vi "GetSettings.vi"(8 "error in (no error)":errorcluster, 10 "SettingsToRetrieve":variant, 11 "NHRDCPower in":refnum<class "NHRDCPower.lvclass">) -> (0 "error out":errorcluster, 2 "RetrievedSettings":variant, 3 "NHRDCPower Out":refnum<class "NHRDCPower.lvclass">)   [LabVIEW 2018, in "AcPwrPlugins.lvlib" / "NHRDCPower.lvclass"]
doc: "This VI retrieves a boolean status to see if the instrument can conduct measurements while the device is changing modes or turning off and on."
uses:
  NHRDCPower.lvclass
  C:/Users/ico/Documents/Projects/NistPluggableModules/AcPwr/AcPwrPlugins/AcPwrBaseClass/AcPwrBase.lvclass
  AcPwrBaseClass/AcPwrBase.lvclass/AcPwrBase.ctl
  AcPwrBaseClass/TypeDefs/BaseMeasurements.ctl
  ChromaAcLoad/TypeDefs/MeasurementType.ctl
  AcPwrBaseClass/Accessors/Read BaseConfig.vi
  AcPwrModule/AcPwrModule.lvlib
  ChromaAcLoad/ChromaAcLoad.lvclass
  AcPwrBaseClass/AcPwrBase.lvclass
panel:
  out "Boolean":bool=TRUE
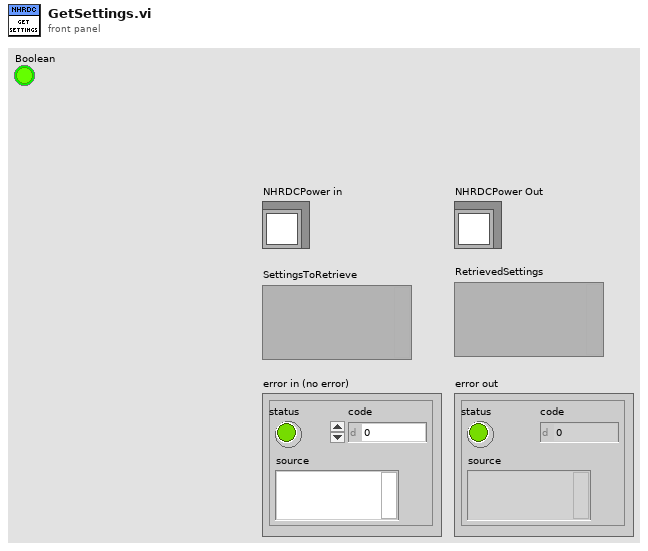
[diagram p1: front panel]
types:
  T1 = typedef "AcPwrPlugins.lvlib/AcPwrBase.lvclass/BaseMeasurements.ctl" = cluster{"Handle":string, "Name":string, "Enabled":bool, "Measurement Value":dbl, "btnMeasFetch":bool, "Chroma Hold Peak Current Measurement":bool, "Chroma Measurement Type":T2, "Chroma Protection Status String":string, "NHRDC Fetch Method":i32, "NHRDC Fetch Time (s)":sgl, "NHRDC Measurement Type":i32, "NHRGridSim Measurement Type ":enum16{"Average Current", "Max Current", "Min Current", "Average Voltage", "Max Voltage", "Min Voltage", "Average True Power", "Max True Power", "Min True Power", "Average Apparent Power", "Max Apparent Power", "Min Apparent Power", "Power Factor", "Crest Factor"}, "NHRGridSim Phase ":i32, "PPS Measurement Type ":enum16{"Voltage RMS L-N", "Voltage RMS L-L", "Frequency", "Current RMS", "Current Peak", "Crest Factor", "Power Factor", "Power VA", "Real Power"}, "PPS Channel Name":enum16{"A", "B", "C"}}[]
  T2 = typedef "AcPwrPlugins.lvlib/ChromaAcLoad.lvclass/MeasurementType.ctl" = enum16{"Voltage (Vrms or V)", "Current (Arms or A)", "Power (W)", "Peak Voltage (V)", "Peak Current (A)", "Peak Power (W)", "Frequency (Hz)", "Resistance (Ohms)", "Voltage Overshoot (V)", "Positive Peak Current (A)", "Voltage Undershoot (V)", "Negative Peak Current (A)", "Apparent Power (VA)", "Reacitive Power (VAR)", "Voltage THD", "Power Factor", "Current's Crest Factor"}
  T3 = typedef "AcPwrPlugins.lvlib/AcPwrBase.lvclass/BaseConfig.ctl" = cluster{"Frequency":dbl, "FrequencyRange":dbl[], "Phases":T4[], "Name":string, "Chroma":T5, "NHRDC":T6, "PPS":T7}
  T4 = typedef "AcPwrPlugins.lvlib/AcPwrBase.lvclass/Phase.ctl" = cluster{"Name":string, "Enabled":bool, "VoltageLevel":dbl, "Handle":string, "VoltageRange":dbl[], "Connected":bool, "CurrentLimit":dbl, "Waveform":string}
  T5 = typedef "AcPwrPlugins.lvlib/ChromaAcLoad.lvclass/DeviceProperties.ctl" = cluster{"Configuration Mode":enum16{"Constant Voltage (DC)", "Constant Power (DC)", "Constant Power (AC)", "Constant Current (DC)", "Constant Current (AC)", "Constant Resistance (DC)", "Constant Resistance (AC)", "Rectified Mode (DC)", "Inrush (AC)", "RLC CP (AC)", "RLC (AC)"}, "Phases":cluster{"Handle":string, "Name":string, "Phase Select":i32, "Instrument Options":string, "id query (T)":bool, "reset device (T)":bool, "Load Short Circuited":bool, "Line Synchronization":bool, "Load Current (A/Arms)":dbl, "Load Voltage (V/Vrms)":dbl, "Load Power (W)":dbl, "Load Resistance (Ohms)":dbl, "Load Current Peak Limit (A)":dbl, "Load Current Limit (A/Arms)":dbl, "Load Power Limit (W)":dbl, "Synch Frequency (Hz)":dbl, "Priority":enum16{"CF Only", "PF Only", "Both (CF)", "Both (PF)"}, "Crest Factor":dbl, "Power Factor":dbl, "Slew Rate":cluster{"Rise Slew Rate (A/ms)":i32, "Fall Slew Rate (A/ms)":i32}, "LC/RLC Mode":cluster{"Capacitance (uF)":i32, "Inductance (uH)":i32, "Series Resistance (Ohm)":dbl, "Parallel Resistance (Ohm)":dbl}, "Timing":cluster{"TimingOn":enum16{""}, "Hours":u32, "Minutes":u32, "Seconds":dbl, "CutoffVoltage":dbl}, "Connected":bool}[]}
  T6 = typedef "AcPwrPlugins.lvlib/NHRDCPower.lvclass/Device(s)Settings.ctl" = cluster{"Handle":string, "Name":string, "id query (Yes)":bool, "reset device (Yes)":bool, "Connected":bool, "Voltage Range (V)":dbl[], "Timing":cluster{"TimingOn":enum16{""}, "Hours":u32, "Minutes":u32, "Seconds":dbl, "CutoffVoltage":dbl}, "Initial Battery Detect Voltage (0)":sgl, "SafetySettings":cluster{"SetWatchDog":bool, "Voltage (V)":sgl, "Current (A)":sgl, "Power (W)":sgl, "Voltage Delay (s)":sgl, "Current Delay (s)":sgl, "Power Delay (s)":sgl}, "Options String":string, "Aperture Time (s)":sgl, "operating state (Off)":i32, "OutputSettings":cluster{"Voltage (V)":sgl, "Current (A)":sgl, "Resistance (Ohms)":sgl, "Power (W)":sgl, "Enable Voltage":bool, "Enable Current":bool, "Enable Resistance":bool, "Enable Power":bool, "Delay After (s)":sgl, "Wait Value (V, A, W)":sgl, "Enable Wait":bool, "Wait on Value":i32}[], "SlewRate":cluster{"Set Voltage Rate V/S":sgl, "Set Current Rate A/S":sgl, "Set Resistance Rate R/S":sgl, "Set Power Rate W/S":sgl}}[]
  T7 = typedef "AcPwrPlugins.lvlib/PacificPowerSource.lvclass/DeviceSettings.ctl" = cluster{"Handle":string, "Connected":bool, "Clear Device (F)":bool, "btnIdQuery":bool, "btnReset":bool, "Program #":cluster{"Phase B (Degrees)":i32, "Waveform A (1: Sine)":i32, "Voltage Level (Va)":dbl, "Program Number (0)":i32, "Voltage Level (Vb) ":dbl, "Form (3: Three)":u16, "Coupling  (0: Direct)":u16, "Frequency (45Hz)":dbl, "Current Limit (40A)":dbl, "Phase C (Degrees)":i32, "Voltage Level (Vc)":dbl, "Waveform B (1: Sine)":i32, "Waveform C (1: Sine)":i32}[], "Impedance Parameters (off, 0.00)":cluster{"State":bool, "Impedance":dbl}, "Transient Execution (F)":bool, "OutputEnabled":bool, "Source Range":cluster{"Frequency Minimum (45 Hz)":dbl, "Frequency Maximum (1200 Hz)":dbl, "Voltage Maximum (V)":dbl, "Voltage Minimum (V)":dbl, "Range Control (0: Auto)":u16, "Initial Voltage (0V)":u16, "Frequency Range (600Hz)":u16}, "Port Type":enum16{"GPIB", "Serial"}}[]
  T8 = typedef "AcPwrModule.lvlib/clBroadcastEvents.ctl" = cluster{"DidInit":refnum<user-event>, "StatusUpdate":refnum<user-event>, "ErrorReport":refnum<user-event>, "DidStop":refnum<user-event>, "PathToINI":refnum<user-event>, "Measurements":refnum<user-event>, "LoadConfigFile":refnum<user-event>, "GetSettings":refnum<user-event>, "SetSettings":refnum<user-event>, "GetType&ID":refnum<user-event>, "GotSettings":refnum<user-event>}
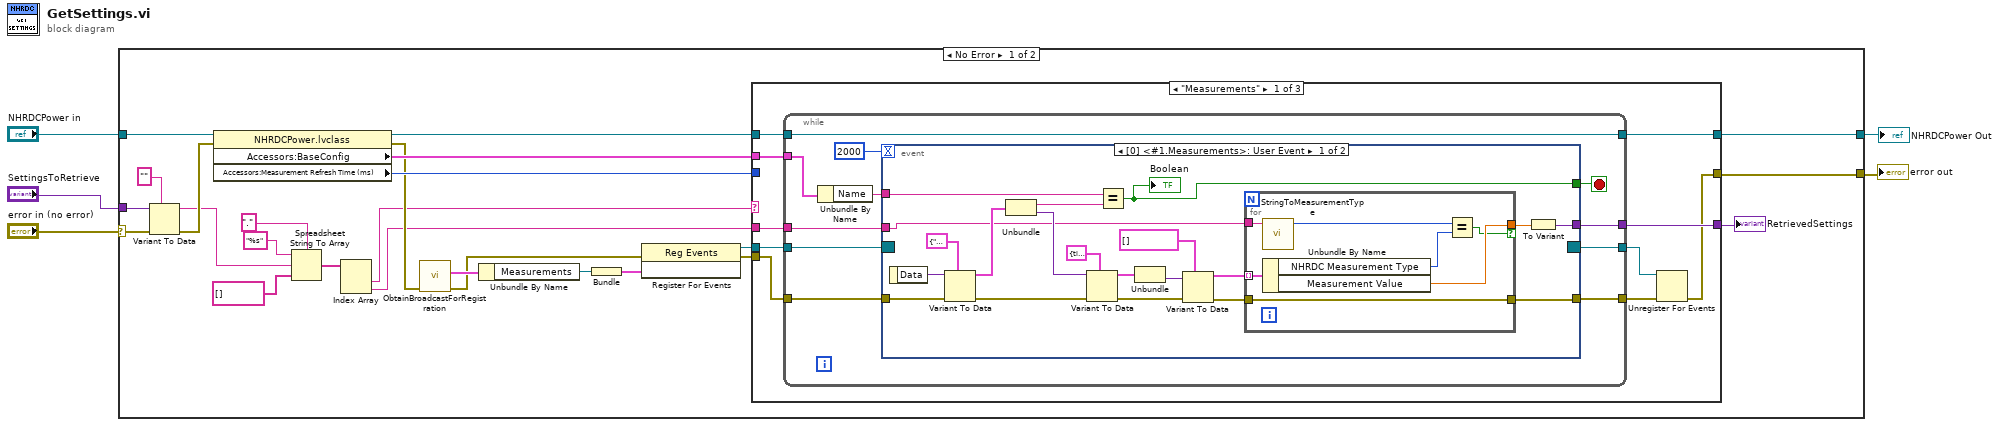
[diagram p0: block diagram]
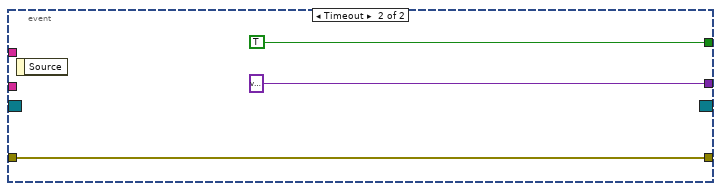
[diagram p2: hidden frame]
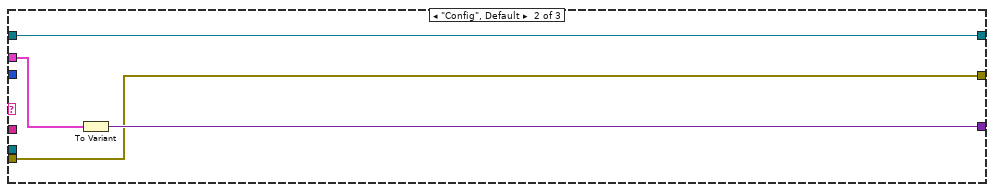
[diagram p3: hidden frame]
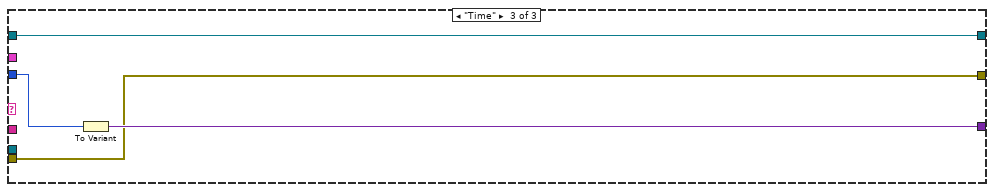
[diagram p4: hidden frame]
diagram:
  n1 = case shown="No Error" "error in (no error)" {
    selector: "error in (no error)" -> [w28 w91]
    tunnel: "NHRDCPower in" -> [w30 w90]
    tunnel: [w21 w91] -> w1
    tunnel: [w22 w90] -> w2
    tunnel: "SettingsToRetrieve" -> [w29 _]
    frame No Error {
      n2 = Variant To Data(error in=w28, type="", Variant=w29) -> (data=w10:string, error out=w27:errorcluster)
      n3 = property class="NHRDCPower.lvclass"(reference=w30, error in=w27) -> (reference out=w23:refnum<class "NHRDCPower.lvclass">, error out=w15:errorcluster, "Accessors:BaseConfig"=w26:T3, "Accessors:Measurement Refresh Time (ms)"=w25:u32)
      n4 = Spreadsheet String To Array(delimiter (Tab)=".", format string="%s", spreadsheet string=w10, array type (2D Dbl)=string[] []) -> (array=w8:string[])
      n5 = Index Array(array=w8) -> (element #1=w7:string, element #2=w6:string)  [unwired: 2 in]
      n6 = call "ObtainBroadcastForRegistration.vi"("error in (no error)"=w15) -> ("error out"=w16:errorcluster, "clBroadcastEvents"=w19:T8)  [unwired: 9 in]
      n7 = Unbundle By Name(w19) -> ("Measurements"=w20:refnum<user-event>)
      n8 = Bundle("Measurements"=w20) -> (w18:cluster{"Measurements":refnum<user-event>})  [unwired: 1 in]
      n9 = register-events(error in=w16, w18) -> (reference out=w17:refnum<event-registration>, error out=w14:errorcluster)  [unwired: 1 in]
      n10 = case shown="\"Measurements\"" w7 {
        tunnel: [w39 w85 w89] -> w13
        tunnel: w26 -> [w32 w82 _]
        tunnel: w25 -> [_ _ w86]
        tunnel: w23 -> [w38 w84 w88]
        tunnel: [w37 w84 w88] -> w22
        tunnel: w14 -> [w40 w83 w87]
        tunnel: [w34 w83 w87] -> w21
        tunnel: w17 -> [w36 _ _]
        tunnel: w6 -> [w31 _ _]
        frame "Measurements" {
          n11 = while {
            tunnel: w36 -> [w51]
            tunnel: [w50] -> w39
            tunnel: w40 -> [w46]
            tunnel: w38 -> [w47]
            tunnel: [w47] -> w37
            tunnel: [w45] -> w35
            tunnel: [w44] -> w33
            tunnel: w32 -> [w43]
            tunnel: w31 -> [w41]
            stop <- w49 stop-if-true
            n12 = Unbundle By Name(w43) -> ("Name"=w42:string)
            n13 = event shown="[0] <#1.Measurements>: User Event" {
              selector: w51 -> [_ _]
              dyn-events: [_ _] -> w45
              timeout: 2000 -> [_ _]
              tunnel: [w56 variant ("Data")] -> w50
              tunnel: [w65 TRUE] -> w49
              tunnel: w46 -> [w71 w79]
              tunnel: [w54 w79] -> w44
              tunnel: w42 -> [w66 _]
              tunnel: w41 -> [w52 _]
              event User Event {
                n14 = event-data() -> ("Data"=w70:variant)  [unwired: 1 in]
                n15 = Variant To Data(error in=w71, type=cluster{string, "Data":variant} {"", "Data"=variant}, Variant=w70) -> (data=w68:cluster{string, "Data":variant}, error out=w62:errorcluster)
                n16 = Unbundle(w68) -> (w67:string, "Data"=w61:variant)
                n17 = Variant To Data(error in=w62, type=cluster{timestamp, "Data":variant} {timestamp(0 s since 1904-01-01), "Data"=variant}, Variant=w61) -> (data=w64:cluster{timestamp, "Data":variant}, error out=w59:errorcluster)
                n18 = Equal?(x=w66, y=w67) -> (x = y?=w65:bool)
                "Boolean" <- w65
                n19 = Unbundle(w64) -> ("Data"=w60:variant)  [unwired: 1 out]
                n20 = Variant To Data(error in=w59, type=T1 [] ("BaseMeasurements"), Variant=w60) -> (data=w57:T1, error out=w55:errorcluster)
                n21 = for {
                  tunnel: w57 -> [w77] mode=indexing
                  tunnel: w55 -> [w78]
                  tunnel: [w78] -> w54
                  tunnel: [w76] -> w53 if=w72
                  tunnel: w52 -> [w75]
                  n22 = call "StringToMeasurementType.vi"("String"=w75) -> ("Measurement Type"=w74:i32)  [unwired: 10 in]
                  n23 = Unbundle By Name(w77) -> ("NHRDC Measurement Type"=w73:i32, "Measurement Value"=w76:dbl)
                  n24 = Equal?(x=w74, y=w73) -> (x = y?=w72:bool)
                }
                n25 = To Variant(anything=w53) -> (Variant=w56:variant)
              }
              event Timeout {
                n26 = event-data() -> ()  [unwired: 1 in, 1 out]
              }
            }
          }
          n27 = Unregister For Events(event registration refnum=w35, error in=w33) -> (error out=w34:errorcluster)
        }
        frame "Config", Default {
          n28 = To Variant(anything=w82) -> (Variant=w85:variant)
        }
        frame "Time" {
          n29 = To Variant(anything=w86) -> (Variant=w89:variant)
        }
      }
      "RetrievedSettings" <- w13
    }
    frame Error {
    }
  }
  "error out" <- w1
  "NHRDCPower Out" <- w2
